vi "Open.vi"(4 "Wait":u32=30000, 6 "Show Panel":bool, 8 "error in (no error)":errorcluster) -> (0 "error out":errorcluster, 3 "LabVIEW Instance":refnum<class "LabVIEW Instance.lvclass">)   [LabVIEW 2014, in "LabVIEW Instance.lvclass"]
uses:
  LabVIEW Instance.lvclass
  LabVIEW Instance.lvclass/LabVIEW Instance.ctl
  <vilib>/Utility/config.llb/Read Key (String).vi
  <vilib>/Utility/config.llb/Read Key (I32).vi
  <vilib>/Utility/config.llb/Read Key (Path).vi
  <vilib>/Utility/config.llb/NI_LVConfig.lvlib
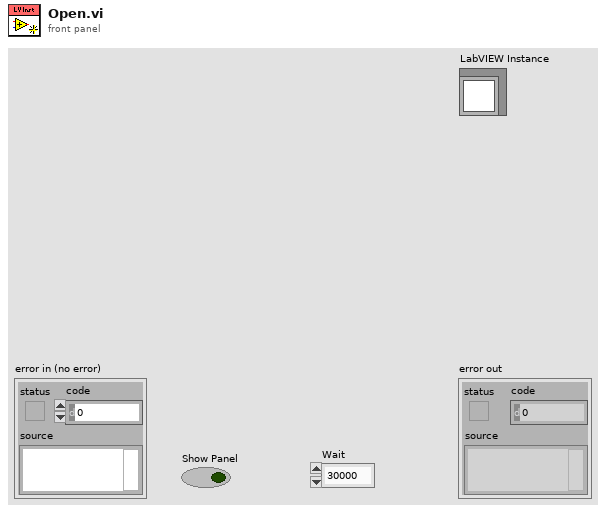
[diagram p1: front panel]
types:
  T1 = typedef "NI_LVConfig.lvlib/Config Data RefNum.ctl" = refnum<k1>
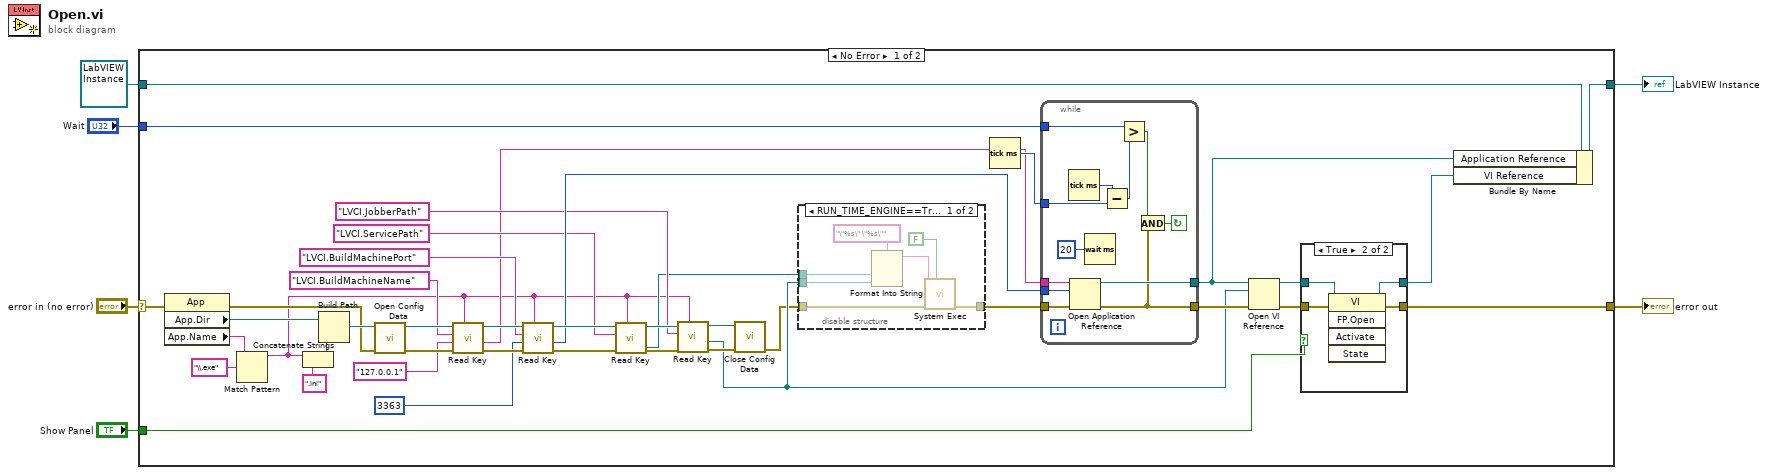
[diagram p0: block diagram]
diagram:
  n1 = case shown="No Error" "error in (no error)" {
    selector: "error in (no error)" -> [w12 w76]
    tunnel: [w41 w76] -> w5
    tunnel: [w45 w75] -> w3
    tunnel: refnum<class "LabVIEW Instance.lvclass"> refnum ("Jobber Proxy in") -> [w48 w75]
    tunnel: "Show Panel" -> [w40 _]
    tunnel: "Wait" -> [w38 _]
    frame No Error {
      n2 = property class="App"(error in=w12) -> (error out=w25:errorcluster, "App.Dir"=w35:path, "App.Name"=w37:string)  [unwired: 1 in, 1 out]
      n3 = Match Pattern(string=w37, regular expression="\\.exe") -> (before substring=w8:string)  [unwired: 1 in, 3 out]
      n4 = Concatenate Strings(w8, ".ini" ("string")) -> (w33:string)
      n5 = Build Path(base path=w35, name or relative path=w33) -> (appended path=w26:path)
      n6 = call <vilib>:"Open Config Data.vi"("error in (no error)"=w25, "configuration file path"=w26) -> ("error out"=w32:errorcluster, "refnum"=w31:T1)  [unwired: 7 in, 1 out]
      n7 = call-poly <vilib>:"Read Key.vi"("section"=w8, "error in (no error)"=w32, "default value"="127.0.0.1", "key"="LVCI.BuildMachineName", "refnum"=w31) -> ("error out"=w29:errorcluster, "value"=w10:string, "refnum out"=w30:T1)  [unwired: 3 in, 1 out]
      n8 = call-poly <vilib>:"Read Key.vi"("section"=w8, "error in (no error)"=w29, "default value"=3363, "key"="LVCI.BuildMachinePort", "refnum"=w30) -> ("error out"=w28:errorcluster, "value"=w20:i32, "refnum out"=w27:T1)  [unwired: 3 in, 1 out]
      n9 = call-poly <vilib>:"Read Key.vi"("section"=w8, "error in (no error)"=w28, "key"="LVCI.ServicePath", "refnum"=w27) -> ("error out"=w17:errorcluster, "value"=w9:path, "refnum out"=w16:T1)  [unwired: 4 in, 1 out]
      n10 = call-poly <vilib>:"Read Key.vi"("section"=w8, "error in (no error)"=w17, "key"="LVCI.JobberPath", "refnum"=w16) -> ("error out"=w19:errorcluster, "value"=w15:path, "refnum out"=w18:T1)  [unwired: 4 in, 1 out]
      n11 = call <vilib>:"Close Config Data.vi"("error in (no error)"=w19, "refnum"=w18) -> ("error out"=w11:errorcluster)  [unwired: 8 in, 1 out]
      n12 = disable-structure shown="RUN_TIME_ENGINE==True" {
        disable-tunnel: w11 -> [w66 w68]
        disable-tunnel: [w63 w68] -> w47
        disable-tunnel: w15 -> [w65 _]
        disable-tunnel: w9 -> [w62 _]
        frame condition #0 {
          n13 = Format Into String(format string="\"%s\" \"%s\"", w62, w65) -> (resulting string=w61:string)  [unwired: 2 in, 1 out]
          n14 = call <vilib>:"System Exec.vi"("wait until completion? (T)"=FALSE, "error in (no error)"=w66, "command line"=w61) -> ("error out"=w63:errorcluster)  [unwired: 5 in, 3 out]
        }
        frame condition #1 (active) {
        }
      }
      n15 = Tick Count (ms)() -> (millisecond timer value=w39:u32)
      n16 = while {
        tunnel: w10 -> [w59]
        tunnel: w20 -> [w58]
        tunnel: [w57] -> w7
        tunnel: w39 -> [w55]
        tunnel: w38 -> [w53]
        tunnel: w47 -> [w60]
        tunnel: [w50] -> w46
        stop <- w52 continue-if-true
        n17 = Tick Count (ms)() -> (millisecond timer value=w56:u32)
        n18 = Open Application Reference(8:w60, 10:w58, 11:w59) -> (0:w50:errorcluster, 3:w57:refnum<vi>)  [unwired: 1 in]
        n19 = Wait (ms)(milliseconds to wait=u32 20) -> ()  [unwired: 1 out]
        n20 = Subtract(x=w56, y=w55) -> (x-y=w54:u32)
        n21 = Greater?(x=w53, y=w54) -> (0:w51:bool)
        n22 = And(x=w51, y=w50) -> (x .and. y?=w52:bool)
      }
      n23 = Open VI Reference(application reference (local)=w7, vi path=w15, error in (no error)=w46) -> (vi reference=w44:refnum<vi>, error out=w42:errorcluster)  [unwired: 3 in]
      n24 = case shown="True" w40 {
        tunnel: w44 -> [w70 w74]
        tunnel: [w70 w73] -> w43
        tunnel: w42 -> [w69 w72]
        tunnel: [w69 w71] -> w41
        frame False {
        }
        frame True {
          n25 = invoke class="VI" method="FP.Open"(reference=w74, error in=w72) -> (reference out=w73:refnum<vi>, error out=w71:errorcluster)  [unwired: 3 in, 3 out]
        }
      }
      n26 = Bundle By Name(cluster=w48, "Application Reference"=w7, "VI Reference"=w43) -> (w45:refnum<class "LabVIEW Instance.lvclass">)
    }
    frame Error {
    }
  }
  "error out" <- w5
  "LabVIEW Instance" <- w3
